vi "GetValuesOfMainMenu.vi"(11 "MainMenu_In":refnum<vi>) -> (0 "ValuesOfMainMenu":T1, 3 "MainMenu_Out":refnum<vi>)   [LabVIEW 2013]
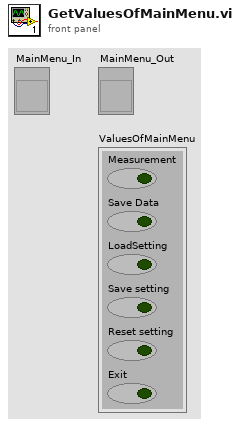
[diagram p1: front panel]
types:
  T1 = cluster{"Measurement":bool, "Save Data":bool, "LoadSetting":bool, "Save setting":bool, "Reset setting":bool, "Exit":bool}
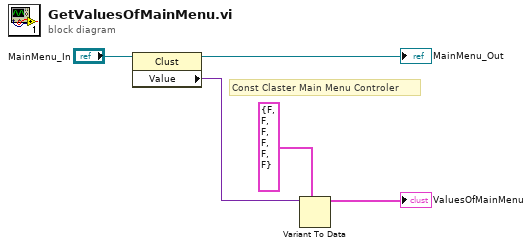
[diagram p0: block diagram]
diagram:
  # "Const Claster Main Menu Controler"
  n1 = property class="Clust"(reference="MainMenu_In") -> (reference out=→"MainMenu_Out":refnum<vi>, "Value"=w1:variant)  [unwired: 1 in, 1 out]
  n2 = Variant To Data(type=T1 {"Measurement"=FALSE, "Save Data"=FALSE, "LoadSetting"=FALSE, "Save setting"=FALSE, "Reset setting"=FALSE, "Exit"=FALSE} ("Main menu"), Variant=w1) -> (data=→"ValuesOfMainMenu":T1)  [unwired: 1 in, 1 out]
